vi "Parse Results (all) (cluster).vi"(6 "Type":T1, 8 "error in (no error)":errorcluster, 11 "Results (Dictionary)":cluster{"key":string, "value":dbl[]}[](array[cluster])) -> (0 "error out":errorcluster, 1 "Label":string[](array[string]), 2 "Data":cluster{"value":dbl[]}[](array[cluster]), 3 "Results (Dictionary)":cluster{"key":string, "value":dbl[]}[](array[cluster]))   [LabVIEW 2019, in "Instrument.Lockin.lvlib" / "Instrument.Lockin.lvclass"]
doc: "This method will search the <b>Results Dictionary</b> for the data specified by <b>Datatype</b> (X, Y, R, Theta, mean).\n\n<b>Data</b> is an array of clusters, of which each element is an array of the matched datatype."
uses:
  Typedefs/Results Type--Enum.ctl
  Instrument.Lockin.lvclass
panel:
  # "UI should call this one"
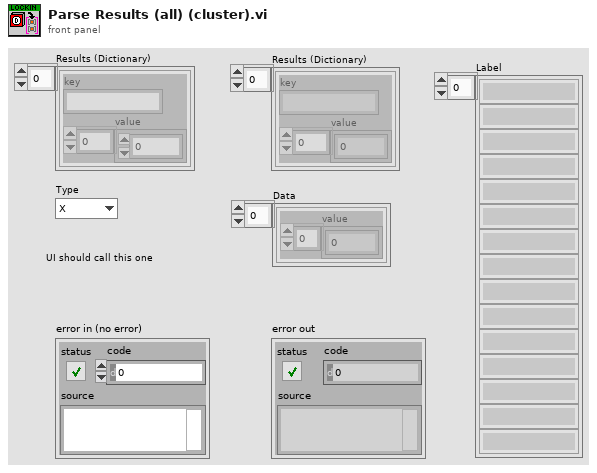
[diagram p1: front panel]
types:
  T1 = typedef "Instrument.Lockin.lvlib/Instrument.Lockin.lvclass/Results Type--Enum.ctl" = enum16{"X", "Y", "R", "Theta", "Mean"}
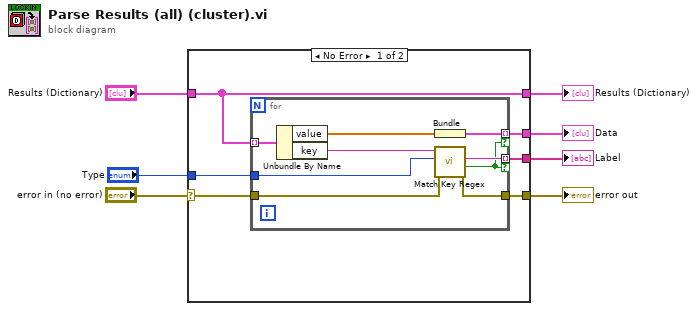
[diagram p0: block diagram]
diagram:
  n1 = case shown="No Error" "error in (no error)" {
    selector: "error in (no error)" -> [w10 w23]
    tunnel: [w13 _] -> w7
    tunnel: "Type" -> [w11 _]
    tunnel: "Results (Dictionary)" -> [w12 w24]
    tunnel: [w9 _] -> w4
    tunnel: [w8 w23] -> w1
    tunnel: [w12 w24] -> w3
    frame No Error {
      n2 = for {
        tunnel: [w20] -> w13 mode=indexing if=w17
        tunnel: w12 -> [w21] mode=indexing
        tunnel: w11 -> [w14]
        tunnel: w10 -> [w16]
        tunnel: [w18] -> w9 mode=indexing if=w17
        tunnel: [w15] -> w8
        n3 = Unbundle By Name(w21) -> ("value"=w22:dbl[], "key"=w19:string)
        n4 = Bundle("value"=w22) -> (w20:cluster{"value":dbl[]})  [unwired: 1 in]
        n5 = call "Match Key Regex.vi"("error in"=w16, "Datatype"=w14, "key in"=w19) -> ("error out"=w15:errorcluster, "Datatype Found?"=w17:bool, "Label out"=w18:string)  [unwired: 5 in, 1 out]
      }
    }
    frame Error {
    }
  }
  "Data" <- w7
  "Results (Dictionary)" <- w3
  "Label" <- w4
  "error out" <- w1
